vi "Exp Avg Sound Level (final value).vi"(0 "scaled signal [EU]":dbl[](array[numeric]) format="%.2f", 1 "exponential mode":enum16{"Slow", "Fast", "Impulse", "Custom"}(ring)=enum."Fast", 2 "time constant [ms]":dbl=125.0 format="%.2f", 5 "sampling frequency [Hz]":dbl=10000.0 format="%.2f", 7 "weighting filter":T1(ring), 9 "type":enum16{"Type 0", "Type 1"}(ring)=enum."Type 1", 11 "channel info":T2={"sensor sensitivity [mV/EU]"=1000.0, "engineering units"=1, "dB reference [EU]"=1.0, "custom label"="EU", "weighting filter"=0, "pregain [dB]"=0.0} {"pregain [dB]" format="%.2f"; "weighting filter" items=["Linear", "A-weighting", "B-weighting", "C-weighting", "ITU-R 468-4", "Dolby", "CCITT", "C-message"]; "dB reference [EU]" format="%^.1e"; "engineering units" items=["custom..."=0, "V"=1, "A"=21, "Pa"=2, "N"=20, "g"=3, "m/s^2"=4, "m/s"=5, "m"=6, "mm/s"=12, "mm"=13, "microns/s"=14, "microns"=15, "in/s^2"=7, "in/s"=8, "in"=9, "mils/s"=10, "mils"=11, "rad/s^2"=16, "rad/s"=17, "rad"=18, "strain"=19]; "sensor sensitivity [mV/EU]" format="%.2f"}, 12 "weighting filter init/cont (init:F)":bool, 13 "exp avg init/cont (init:F)":bool) -> (4 "exp avg sound level [dB EU] (final value)":dbl format="%.2f", 6 "unit label":string, 8 "max freq within tolerances [Hz]":dbl format="%.2f", 10 "actual time constant [ms]":dbl=125.0 format="%.2f", 15 "weighting conflict":bool)   [LabVIEW 2017]
doc: "Computes the exponential averaged sound level of the input signal X, based on the selected exponential averaging mode, and returns the last value of this sound level, expressed in decibels."
uses:
  <vilib>/addons/Sound and Vibration/compatibility/Controls/svl_Channel Info.ctl
  <vilib>/addons/Sound and Vibration/compatibility/Controls/svl_Engineering Units Text Ring.ctl
  <vilib>/addons/Sound and Vibration/compatibility/Controls/svl_Weighting Filter Text Ring.ctl
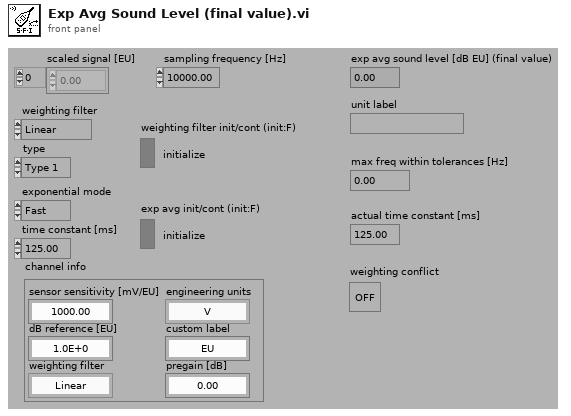
[diagram p1: front panel]
types:
  T1 = enum16{"Linear", "A-weighting", "B-weighting", "C-weighting"}
  T2 = typedef "svl_Channel Info.ctl" = cluster{"sensor sensitivity [mV/EU]":dbl, "engineering units":T3, "dB reference [EU]":dbl, "custom label":string, "weighting filter":T4, "pregain [dB]":dbl}
  T3 = typedef "svl_Engineering Units Text Ring.ctl" = u16
  T4 = typedef "svl_Weighting Filter Text Ring.ctl" = u16
  T5 = cluster{"exponential averaging":dbl, "peak detector":dbl}
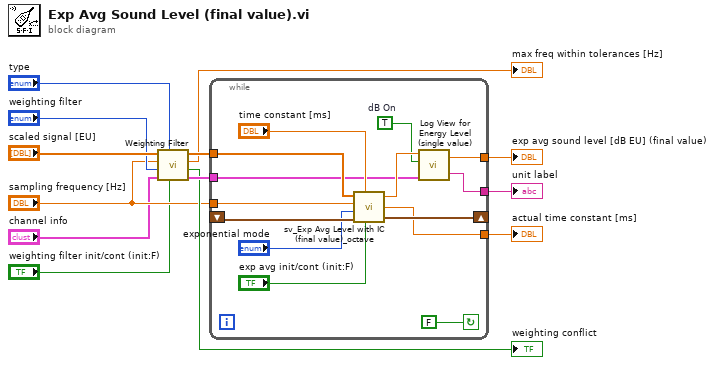
[diagram p0: block diagram]
diagram:
  n1 = call <vilib>:"Weighting Filter.vi"("weighting filter init/cont (init:F)"="weighting filter init/cont (init:F)", "type"="type", "channel info IN"="channel info", "weighting filter"="weighting filter", "sampling frequency [Hz]"="sampling frequency [Hz]", "scaled signal [EU]"="scaled signal [EU]") -> ("channel info OUT"=w9:T2, "weighting conflict"=→"weighting conflict":bool, "max freq within tolerances [Hz]"=→"max freq within tolerances [Hz]":dbl, "weighted signal [EU]"=w10:dbl[])
  n2 = while {
    tunnel: w9 -> [w15]
    tunnel: [w20] -> w11
    tunnel: [w21] -> w12
    tunnel: [w22] -> w13
    tunnel: "sampling frequency [Hz]" -> [w25]
    tunnel: w10 -> [w26]
    shift-left: _ -> [w19]
    shift-right: [w27] -> _
    stop <- FALSE continue-if-true
    w23 = TRUE  # dB On
    n3 = call <vilib>:"sv_Exp Avg Level with IC (final value)_octave.vi"("scaled signal [EU]"=w26, "time constant [ms]"="time constant [ms]", "sampling frequency [Hz]"=w25, "exponential mode"="exponential mode", "init/cont (init:F)"="exp avg init/cont (init:F)", "initial filter state"=w19) -> ("exp avg [EU^2 rms] (final value)"=w24:dbl, "actual time constant [ms]"=w20:dbl, "final filter state"=w27:T5)
    n4 = call <vilib>:"Log View for Energy Level (single value).vi"("channel info"=w15, "dB On (T)"=w23, "energy level [EU^2 rms]"=w24) -> ("unit label"=w21:string, "log view [dB EU]"=w22:dbl)  [unwired: 1 in]
  }
  "exp avg sound level [dB EU] (final value)" <- w13
  "unit label" <- w12
  "actual time constant [ms]" <- w11
